vi "ECS - XNET CAN Interface.vi"() -> ()   [LabVIEW 2015, in "ECS-RT.lvlib"]
uses:
  ECS-RT.lvlib
  Typedefs/MISC/Control Parameters.ctl
  Globals/Calpoint IDs.vi
  <vilib>/xnet/xnet.llb/XNET String To IO Name (Database Alias).vi
  <vilib>/xnet/xnet.llb/XNET Database Close (Database).vi
  <vilib>/xnet/xnet.llb/XNET String To IO Name (Signal).vi
  <vilib>/xnet/xnet.llb/XNET Create Session (Signal Input Single-point).vi
  <vilib>/xnet/xnet.llb/XNET Read (Signal Single-point).vi
  <vilib>/xnet/xnet.llb/XNET Create Session (Signal Output Single-point).vi
  <vilib>/xnet/xnet.llb/XNET Write (Signal Single-point).vi
  <resource>/objmgr/xnet.rc
  <vilib>/addons/Software Calibration Management/_CalPointResources/scm32.dll
  ECS-Shared.lvlib
panel:
  out "XNET Control Params":T1[](array[typedef])
  in  "Wait":u32=2500 caption="[msec]"
  out "error out":errorcluster
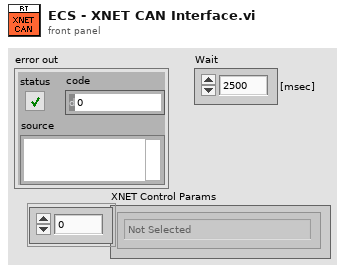
[diagram p1: front panel]
types:
  T1 = typedef "ECS-Shared.lvlib/Control Parameters.ctl" = enum16{"Not Selected", "Pedal Position [%]", "ESTOP", "Sensor1NOx", "Sensor1O2", "Sensor1SupplyStatus", "Sensor1TempStatus", "Sensor1NOxStatus", "Sensor1O2Status", "Sensor1HeaterMode", "Sensor1HeaterCircuit", "Sensor1NOxCircuit", "Sensor1O2Circuit", "Sensor2NOx", "Sensor2O2", "Sensor2SupplyStatus", "Sensor2TempStatus", "Sensor2NOxStatus", "Sensor2O2Status", "Sensor2HeaterMode", "Sensor2HeaterCircuit", "Sensor2NOxCircuit", "Sensor2O2Circuit"}
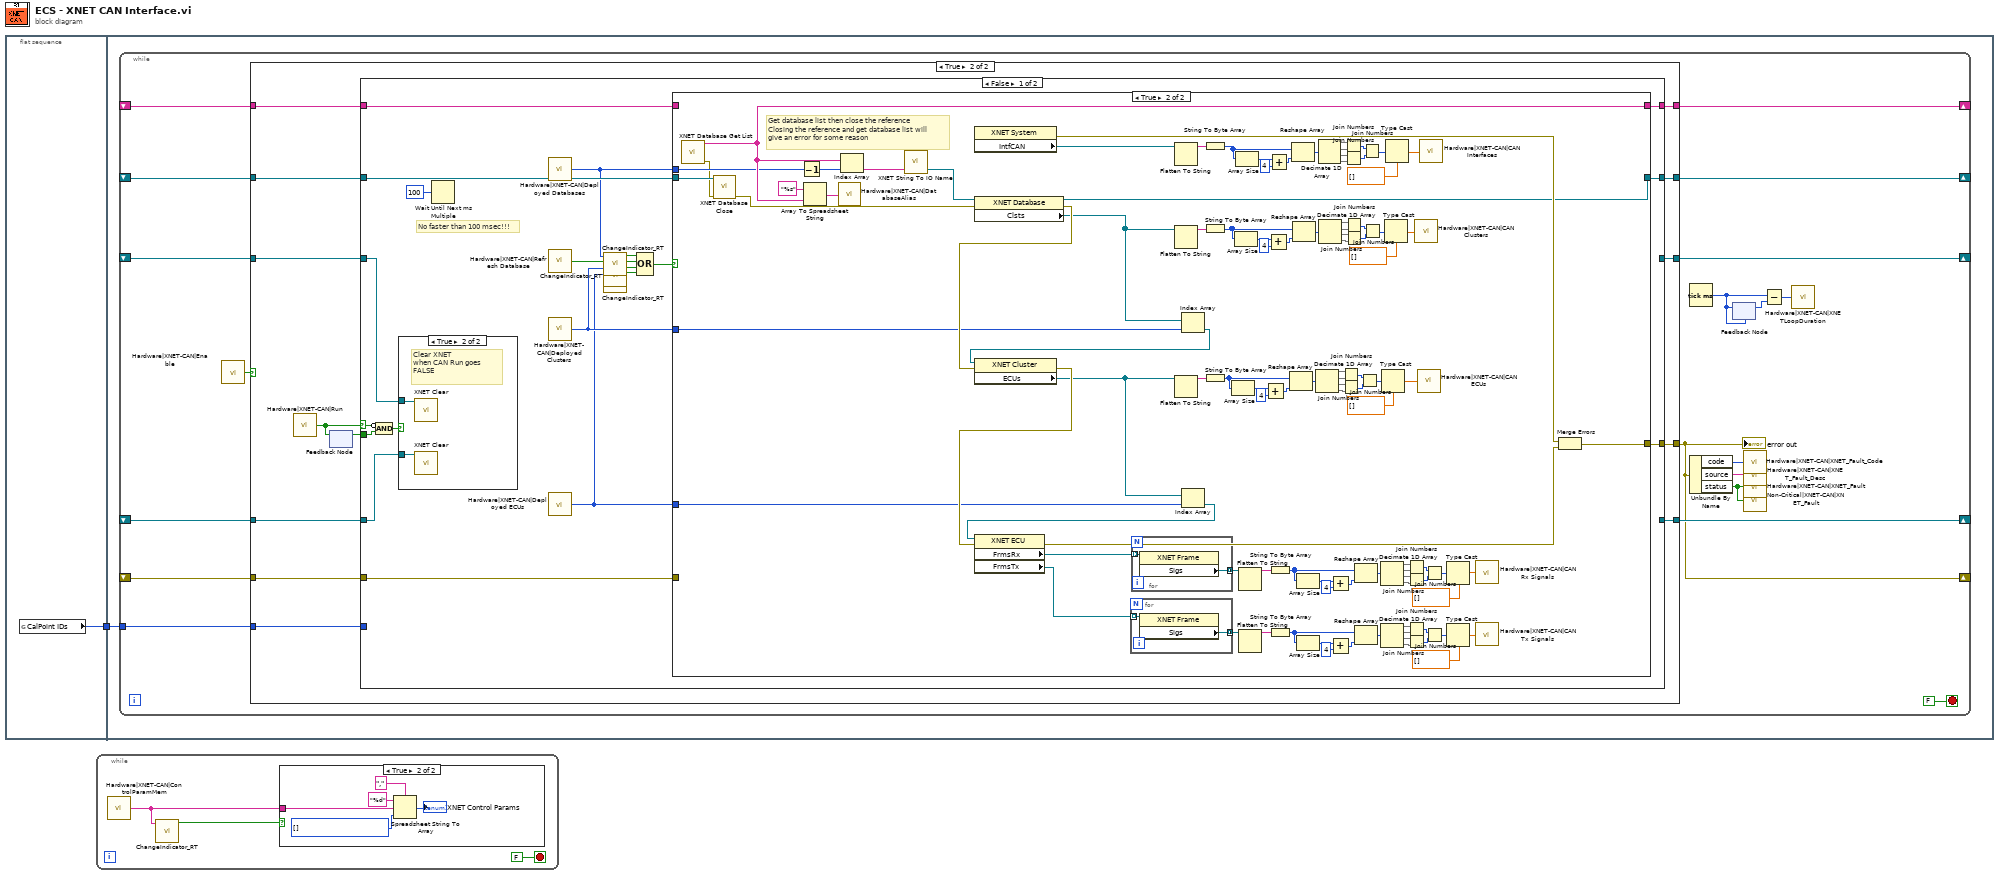
[diagram p0: block diagram]
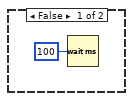
[diagram p2: hidden frame]
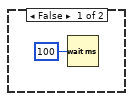
[diagram p3: hidden frame]
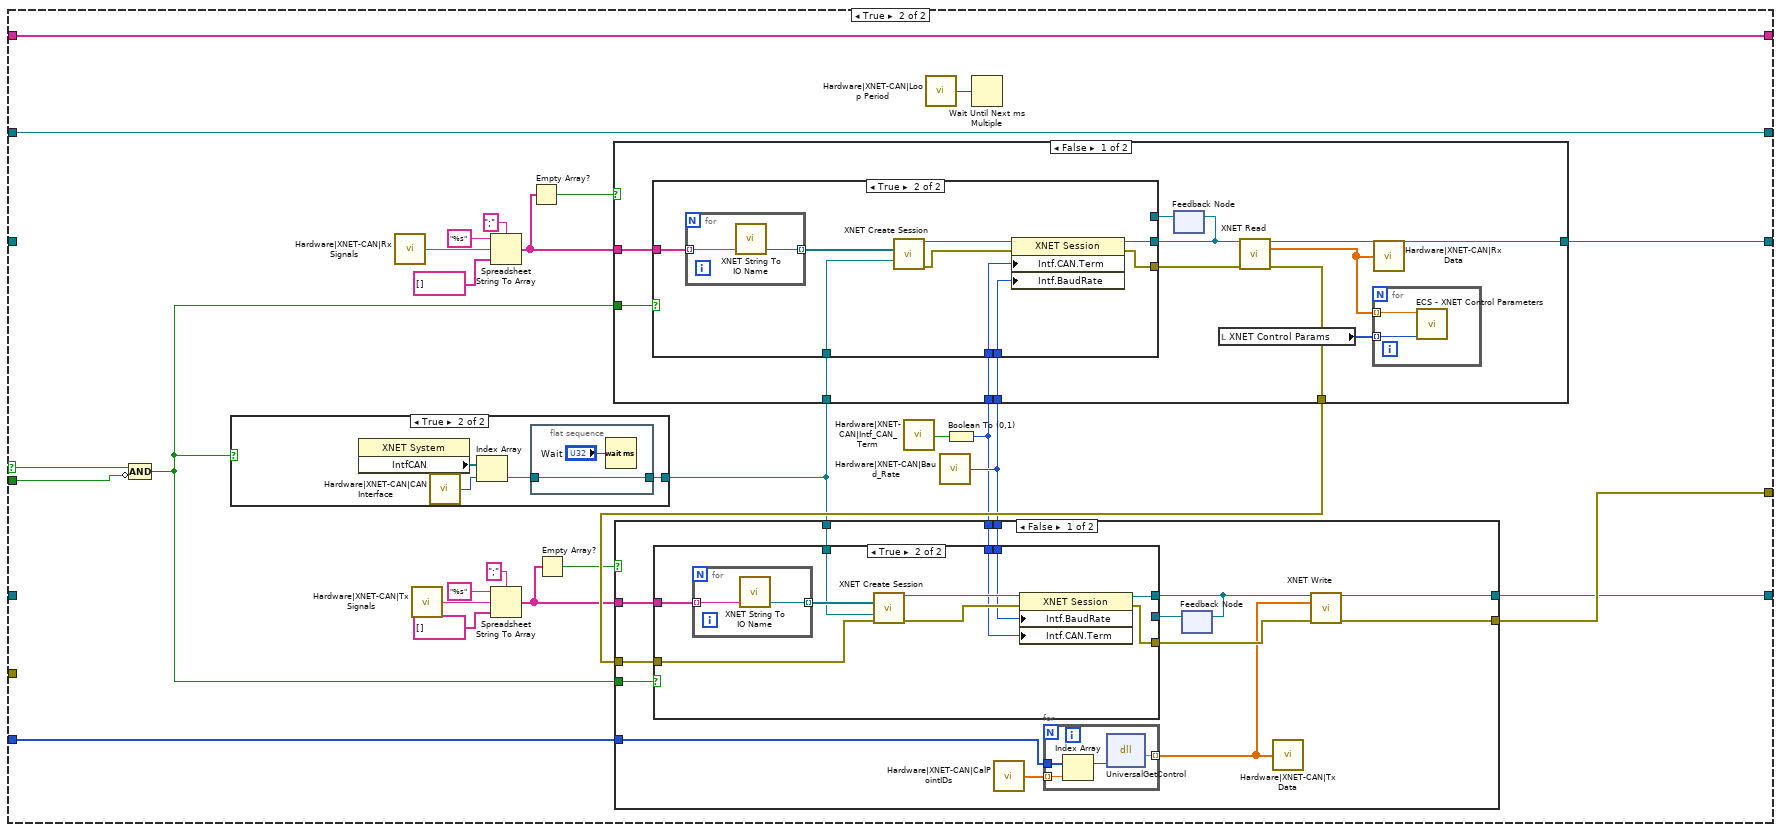
[diagram p6: hidden frame]
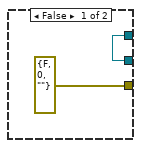
[diagram p8: hidden frame]
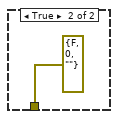
[diagram p9: hidden frame]
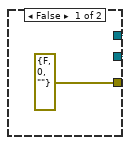
[diagram p10: hidden frame]
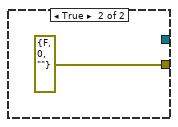
[diagram p11: hidden frame]
diagram:
  n1 = flat-sequence {
    tunnel: [w2] -> w1
    tunnel: w1 -> [w3]
    frame #0 {
      n2 = global read "Calpoint IDs.vi" "CalPoint IDs"() -> (w2:i32[])
    }
    frame #1 {
      n3 = while {
        shift-right: [w21] -> _
        shift-left: _ -> [w19]
        shift-right: [w22] -> _
        shift-left: _ -> [w20]
        shift-right: [w18] -> _
        shift-left: _ -> [w17]
        shift-right: [w11] -> _
        shift-left: _ -> [w10]
        shift-right: [w9] -> _
        shift-left: _ -> [w8]
        tunnel: w3 -> [w7]
        stop <- FALSE stop-if-true
        n4 = call "Hardware|XNET-CAN|Enable"() -> ("Value"=w4:bool)
        n5 = case shown="True" w4 {
          tunnel: [_ w34] -> w22
          tunnel: [_ w33] -> w21
          tunnel: w20 -> [_ w32]
          tunnel: w19 -> [_ w31]
          tunnel: [_ w30] -> w18
          tunnel: w17 -> [_ w29]
          tunnel: [_ w28] -> w11
          tunnel: w10 -> [_ w27]
          tunnel: [_ w26] -> w9
          tunnel: w8 -> [_ w25]
          tunnel: w7 -> [_ w24]
          frame False {
            n6 = Wait (ms)(milliseconds to wait=u32 100) -> ()  [unwired: 1 out]
          }
          frame True {
            n7 = call "Hardware|XNET-CAN|Run"() -> ("Value"=w36:bool)
            n8 = feedback #1() -> (w35:bool)  [unwired: 1 in]
            n9 = feedback-in #1(w36) -> ()
            n10 = case shown="False" w36 {
              selector: w36 -> [w56 w193]
              tunnel: [w51 w180] -> w26
              tunnel: w35 -> [w54 w171]
              tunnel: [_ w177] -> w34
              tunnel: [_ w176] -> w33
              tunnel: w32 -> [w53 _]
              tunnel: w31 -> [w52 _]
              tunnel: [w50 w173] -> w30
              tunnel: w29 -> [w48 w173]
              tunnel: [w49 w170] -> w28
              tunnel: w27 -> [w37 w170]
              tunnel: w25 -> [w38 _]
              tunnel: w24 -> [_ w168]
              frame False {
                # "No faster than 100 msec!!!"
                n11 = Compound Arithmetic op=AND(invert w56, w54) -> (w55:bool)
                n12 = case shown="True" w55 {
                  tunnel: w53 -> [_ w167]
                  tunnel: w52 -> [_ w166]
                  frame False {
                  }
                  frame True {
                    # "Clear XNET\nwhen CAN Run goes FALSE"
                    n13 = call <vilib>:"XNET Clear.vi"("session in"=w166) -> ()  [unwired: 14 in, 1 out]
                    n14 = call <vilib>:"XNET Clear.vi"("session in"=w167) -> ()  [unwired: 14 in, 1 out]
                  }
                }
                n15 = Wait Until Next ms Multiple(millisecond multiple=u32 100) -> ()  [unwired: 1 out]
                n16 = call "Hardware|XNET-CAN|Deployed Databases"() -> ("Value"=w44:i32)
                n17 = call "Hardware|XNET-CAN|Refresh Database"() -> ("Value"=w46:bool)
                n18 = call "Hardware|XNET-CAN|Deployed Clusters"() -> ("Value"=w41:i32)
                n19 = call "Hardware|XNET-CAN|Deployed ECUs"() -> ("Value"=w40:i32)
                n20 = call "ChangeIndicator_RT.vi"("Input"=w44) -> ("Change"=w45:bool)  [unwired: 9 in]
                n21 = call "ChangeIndicator_RT.vi"("Input"=w41) -> ("Change"=w43:bool)  [unwired: 9 in]
                n22 = call "ChangeIndicator_RT.vi"("Input"=w40) -> ("Change"=w42:bool)  [unwired: 9 in]
                n23 = Compound Arithmetic op=OR(w45, w46, w43, w42) -> (w39:bool)
                n24 = case shown="True" w39 {
                  tunnel: w40 -> [_ w159]
                  tunnel: [w59 w158] -> w51
                  tunnel: w41 -> [_ w151]
                  tunnel: [w57 w145] -> w50
                  tunnel: [w58 w144] -> w49
                  tunnel: w48 -> [w57 w143]
                  tunnel: w44 -> [_ w142]
                  tunnel: w38 -> [w59 _]
                  tunnel: w37 -> [w58 _]
                  frame False {
                  }
                  frame True {
                    # "Get database list then close the reference\nClosing the reference and get database list will\ngive an error for some reason"
                    n25 = call <vilib>:"XNET Database Get List.vi"() -> ("array of alias"=w144:string[], "error out"=w60:errorcluster)  [unwired: 13 in, 1 out]
                    n26 = call-poly <vilib>:"XNET Database Close.vi"("database in"=w143, "error in (no error)"=w60) -> ("error out"=w155:errorcluster)  [unwired: 13 in]
                    n27 = Decrement(x=w142) -> (x-1=w61:i32)
                    n28 = Array To Spreadsheet String(array=w144, 3:"%s" ("format string")) -> (spreadsheet string=w63:string)  [unwired: 1 in]
                    n29 = call "Hardware|XNET-CAN|DatabaseAlias"("Value"=w63) -> ()
                    n30 = Index Array(array=w144, index=w61) -> (element=w62:string)
                    n31 = call-poly <vilib>:"XNET String To IO Name.vi"("string"=w62) -> ("XNET Database"=w156:refnum<k21>)  [unwired: 4 out]
                    n32 = property class="XNET System"() -> (error out=w153:errorcluster, "IntfCAN"=w152:refnum<k21>[])  [unwired: 2 in, 1 out]
                    n33 = property class="XNET Database"(reference=w156, error in=w155) -> (reference out=w145:refnum<k21>, error out=w161:errorcluster, "Clsts"=w150:refnum<k21>[])
                    n34 = Flatten To String(anything=w152) -> (data string=w66:string)  [unwired: 3 in, 2 out]
                    n35 = Flatten To String(anything=w150) -> (data string=w81:string)  [unwired: 3 in, 2 out]
                    n36 = Index Array(array=w150, index=w151) -> (element=w149:refnum<k21>)
                    n37 = property class="XNET Cluster"(reference=w149, error in=w161) -> (error out=w160:errorcluster, "ECUs"=w148:refnum<k21>[])  [unwired: 1 out]
                    n38 = Flatten To String(anything=w148) -> (data string=w96:string)  [unwired: 3 in, 2 out]
                    n39 = Index Array(array=w148, index=w159) -> (element=w154:refnum<k21>)
                    n40 = property class="XNET ECU"(reference=w154, error in=w160) -> (error out=w157:errorcluster, "FrmsRx"=w147:refnum<k21>[], "FrmsTx"=w146:refnum<k21>[])  [unwired: 1 out]
                    n41 = for {
                      tunnel: w146 -> [w163] mode=indexing
                      tunnel: [w162] -> w110 mode=concatenating
                      n42 = property class="XNET Frame"(reference=w163) -> ("Sigs"=w162:refnum<k21>[])  [unwired: 1 in, 2 out]
                    }
                    n43 = for {
                      tunnel: w147 -> [w165] mode=indexing
                      tunnel: [w164] -> w111 mode=concatenating
                      n44 = property class="XNET Frame"(reference=w165) -> ("Sigs"=w164:refnum<k21>[])  [unwired: 1 in, 2 out]
                    }
                    n45 = String To Byte Array(string=w66) -> (unsigned byte array=w75:u8[])
                    n46 = String To Byte Array(string=w81) -> (unsigned byte array=w90:u8[])
                    n47 = String To Byte Array(string=w96) -> (unsigned byte array=w105:u8[])
                    n48 = Array Size(array=w105) -> (size(s)=w106:i32)
                    n49 = Array Size(array=w90) -> (size(s)=w91:i32)
                    n50 = Array Size(array=w75) -> (size(s)=w76:i32)
                    n51 = Flatten To String(anything=w111) -> (data string=w141:string)  [unwired: 3 in, 2 out]
                    n52 = Flatten To String(anything=w110) -> (data string=w112:string)  [unwired: 3 in, 2 out]
                    n53 = Add(x=w106, y=4) -> (x+y=w107:i32)
                    n54 = Add(x=w91, y=4) -> (x+y=w92:i32)
                    n55 = Add(x=w76, y=4) -> (x+y=w77:i32)
                    n56 = String To Byte Array(string=w141) -> (unsigned byte array=w132:u8[])
                    n57 = String To Byte Array(string=w112) -> (unsigned byte array=w121:u8[])
                    n58 = Reshape Array(w105, w107) -> (w104:u8[])
                    n59 = Reshape Array(w75, w77) -> (w74:u8[])
                    n60 = Reshape Array(w90, w92) -> (w89:u8[])
                    n61 = Array Size(array=w132) -> (size(s)=w131:i32)
                    n62 = Array Size(array=w121) -> (size(s)=w122:i32)
                    n63 = Decimate 1D Array(w104) -> (w109:u8[], w97:u8[], w98:u8[], w99:u8[])
                    n64 = Decimate 1D Array(w74) -> (w79:u8[], w67:u8[], w68:u8[], w69:u8[])
                    n65 = Decimate 1D Array(w89) -> (w94:u8[], w82:u8[], w83:u8[], w84:u8[])
                    n66 = Add(x=w131, y=4) -> (x+y=w130:i32)
                    n67 = Add(x=w122, y=4) -> (x+y=w123:i32)
                    n68 = Join Numbers(hi=w109, lo=w97) -> ((hi.lo)=w100:u16[])
                    n69 = Join Numbers(hi=w98, lo=w99) -> ((hi.lo)=w101:u16[])
                    n70 = Join Numbers(hi=w79, lo=w67) -> ((hi.lo)=w70:u16[])
                    n71 = Join Numbers(hi=w68, lo=w69) -> ((hi.lo)=w71:u16[])
                    n72 = Join Numbers(hi=w94, lo=w82) -> ((hi.lo)=w85:u16[])
                    n73 = Join Numbers(hi=w83, lo=w84) -> ((hi.lo)=w86:u16[])
                    n74 = Reshape Array(w132, w130) -> (w133:u8[])
                    n75 = Reshape Array(w121, w123) -> (w120:u8[])
                    n76 = Join Numbers(hi=w100, lo=w101) -> ((hi.lo)=w102:u32[])
                    n77 = Join Numbers(hi=w70, lo=w71) -> ((hi.lo)=w72:u32[])
                    n78 = Join Numbers(hi=w85, lo=w86) -> ((hi.lo)=w87:u32[])
                    n79 = Decimate 1D Array(w133) -> (w128:u8[], w140:u8[], w139:u8[], w138:u8[])
                    n80 = Decimate 1D Array(w120) -> (w125:u8[], w113:u8[], w114:u8[], w115:u8[])
                    n81 = Type Cast(type=sgl[] [], x=w102) -> (*(type *) &x=w95:sgl[])
                    n82 = Type Cast(type=sgl[] [], x=w87) -> (*(type *) &x=w80:sgl[])
                    n83 = Type Cast(type=sgl[] [], x=w72) -> (*(type *) &x=w65:sgl[])
                    n84 = Join Numbers(hi=w128, lo=w140) -> ((hi.lo)=w137:u16[])
                    n85 = Join Numbers(hi=w139, lo=w138) -> ((hi.lo)=w136:u16[])
                    n86 = Join Numbers(hi=w125, lo=w113) -> ((hi.lo)=w116:u16[])
                    n87 = Join Numbers(hi=w114, lo=w115) -> ((hi.lo)=w117:u16[])
                    n88 = call "Hardware|XNET-CAN|CAN Clusters"("Value"=w80) -> ()
                    n89 = call "Hardware|XNET-CAN|CAN ECUs"("Value"=w95) -> ()
                    n90 = call "Hardware|XNET-CAN|CAN Interfaces"("Value"=w65) -> ()
                    n91 = Join Numbers(hi=w137, lo=w136) -> ((hi.lo)=w135:u32[])
                    n92 = Join Numbers(hi=w116, lo=w117) -> ((hi.lo)=w118:u32[])
                    n93 = Type Cast(type=sgl[] [], x=w135) -> (*(type *) &x=w127:sgl[])
                    n94 = Type Cast(type=sgl[] [], x=w118) -> (*(type *) &x=w126:sgl[])
                    n95 = call "Hardware|XNET-CAN|CAN Rx Signals"("Value"=w127) -> ()
                    n96 = call "Hardware|XNET-CAN|CAN Tx Signals"("Value"=w126) -> ()
                    n97 = Merge Errors(w153, w157) -> (w158:errorcluster)
                  }
                }
              }
              frame True {
                n98 = Compound Arithmetic op=AND(w193, invert w171) -> (w172:bool)
                n99 = case shown="True" w172 {
                  tunnel: [_ w195] -> w181
                  frame False {
                  }
                  frame True {
                    n100 = property class="XNET System"() -> ("IntfCAN"=w197:refnum<k21>[])  [unwired: 2 in, 2 out]
                    n101 = call "Hardware|XNET-CAN|CAN Interface"() -> ("Value"=w198:u8)
                    n102 = Index Array(array=w197, index=w198) -> (element=w196:refnum<k21>)
                    n103 = flat-sequence {
                      tunnel: w196 -> [w199]
                      tunnel: [w199] -> w195
                      frame #0 {
                        n104 = Wait (ms)(milliseconds to wait="Wait") -> ()  [unwired: 1 out]
                      }
                    }
                  }
                }
                n105 = call "Hardware|XNET-CAN|Rx Signals"() -> ("Value"=w184:string)
                n106 = call "Hardware|XNET-CAN|Tx Signals"() -> ("Value"=w191:string)
                n107 = Spreadsheet String To Array(delimiter (Tab)=";", format string="%s", spreadsheet string=w184, array type (2D Dbl)=string[] [] ("CAN Signals 2")) -> (array=w182:string[])
                n108 = Spreadsheet String To Array(delimiter (Tab)=";", format string="%s", spreadsheet string=w191, array type (2D Dbl)=string[] [] ("CAN Signals 2")) -> (array=w188:string[])
                n109 = Empty Array?(array=w182) -> (empty?=w183:bool)
                n110 = Empty Array?(array=w188) -> (empty?=w189:bool)
                n111 = call "Hardware|XNET-CAN|Intf_CAN_Term"() -> ("Value"=w175:bool)
                n112 = call "Hardware|XNET-CAN|Loop Period"() -> ("Value"=w169:u32)
                n113 = call "Hardware|XNET-CAN|Baud_Rate"() -> ("Value"=w187:u32)
                n114 = Boolean To (0,1)(Boolean=w175) -> (0, 1=w174:i16)
                n115 = case shown="False" w183 {
                  tunnel: w187 -> [w212 _]
                  tunnel: w172 -> [w208 _]
                  tunnel: w182 -> [w207 _]
                  tunnel: w181 -> [w206 _]
                  tunnel: [w205 errorcluster {"status"=FALSE, "code"=0, "source"=""} ("error out")] -> w194
                  tunnel: [w204 _] -> w176
                  tunnel: w174 -> [w203 _]
                  frame False {
                    n116 = feedback #2() -> (w209:refnum<k21>)  [unwired: 1 in]
                    n117 = case shown="True" w208 {
                      tunnel: w212 -> [_ w223]
                      tunnel: [errorcluster {"status"=FALSE, "code"=0, "source"=""} ("error out") w222] -> w211
                      tunnel: [w216 w221] -> w210
                      tunnel: w209 -> [w216 _]
                      tunnel: w207 -> [_ w220]
                      tunnel: w206 -> [_ w219]
                      tunnel: w203 -> [_ w217]
                      frame False {
                      }
                      frame True {
                        n118 = for {
                          tunnel: [w226] -> w225 mode=indexing
                          tunnel: w220 -> [w227] mode=indexing
                          n119 = call-poly <vilib>:"XNET String To IO Name.vi"("string"=w227) -> ("XNET Signal"=w226:refnum<k21>)  [unwired: 4 out]
                        }
                        n120 = call-poly <vilib>:"XNET Create Session.vi"("signal list"=w225, "interface"=w219) -> ("session out"=w224:refnum<k21>, "error out"=w218:errorcluster)  [unwired: 1 in, 11 out]
                        n121 = property class="XNET Session"(reference=w224, error in=w218, "Intf.CAN.Term"=w217, "Intf.BaudRate"=w223) -> (reference out=w221:refnum<k21>, error out=w222:errorcluster)
                      }
                    }
                    n122 = feedback-in #2(w210) -> ()
                    n123 = local read "XNET Control Params"() -> (w202:T1[])
                    n124 = call-poly <vilib>:"XNET Read.vi"("session in"=w210, "error in (no error)"=w211) -> ("session out"=w204:refnum<k21>, "data"=w201:dbl[], "error out"=w205:errorcluster)  [unwired: 11 in]
                    n125 = for {
                      tunnel: w202 -> [w213] mode=indexing
                      tunnel: w201 -> [w214] mode=indexing
                      n126 = call "ECS - XNET Control Parameters.vi"("XNET Control Parameters"=w213, "Rx Data"=w214) -> ()  [unwired: 10 in]
                    }
                    n127 = call "Hardware|XNET-CAN|Rx Data"("Value"=w201) -> ()
                  }
                  frame True {
                  }
                }
                n128 = case shown="False" w189 {
                  tunnel: [w241 errorcluster {"status"=FALSE, "code"=0, "source"=""} ("error out")] -> w180
                  tunnel: w172 -> [w239 _]
                  tunnel: w188 -> [w238 _]
                  tunnel: w187 -> [w237 _]
                  tunnel: w181 -> [w235 _]
                  tunnel: w194 -> [w234 _]
                  tunnel: [w233 _] -> w177
                  tunnel: w174 -> [w232 _]
                  tunnel: w168 -> [w229 _]
                  frame False {
                    n129 = call "Hardware|XNET-CAN|CalPointIDs"() -> ("Value"=w231:sgl[])
                    n130 = for {
                      tunnel: w229 -> [w246]
                      tunnel: [w245] -> w230 mode=indexing
                      tunnel: w231 -> [w243] mode=indexing
                      n131 = Index Array(array=w246, index=w243) -> (element=w244:i32)
                      n132 = dll-call lib="C:/Program Files (x86)/National Instruments/LabVIEW 2015/vi.lib/addons/Software Calibration Management/_CalPointResources/scm*.*" fn="UniversalGetControl"("ID"=w244) -> ("return type"=w245:sgl)  [unwired: 4 in, 2 out]
                    }
                    n133 = feedback #3() -> (w240:refnum<k21>)  [unwired: 1 in]
                    n134 = case shown="True" w239 {
                      tunnel: [w248 w256] -> w242
                      tunnel: w240 -> [w248 _]
                      tunnel: [errorcluster {"status"=FALSE, "code"=0, "source"=""} ("error out") w254] -> w236
                      tunnel: w237 -> [_ w253]
                      tunnel: w238 -> [_ w252]
                      tunnel: w235 -> [_ w251]
                      tunnel: w234 -> [_ w250]
                      tunnel: w232 -> [_ w249]
                      frame False {
                      }
                      frame True {
                        n135 = for {
                          tunnel: [w259] -> w258 mode=indexing
                          tunnel: w252 -> [w260] mode=indexing
                          n136 = call-poly <vilib>:"XNET String To IO Name.vi"("string"=w260) -> ("XNET Signal"=w259:refnum<k21>)  [unwired: 4 out]
                        }
                        n137 = call-poly <vilib>:"XNET Create Session.vi"("signal list"=w258, "interface"=w251, "error in (no error)"=w250) -> ("session out"=w257:refnum<k21>, "error out"=w255:errorcluster)  [unwired: 11 out]
                        n138 = property class="XNET Session"(reference=w257, error in=w255, "Intf.BaudRate"=w253, "Intf.CAN.Term"=w249) -> (reference out=w256:refnum<k21>, error out=w254:errorcluster)
                      }
                    }
                    n139 = feedback-in #3(w242) -> ()
                    n140 = call "Hardware|XNET-CAN|Tx Data"("Value"=w230) -> ()
                    n141 = call-poly <vilib>:"XNET Write.vi"("session in"=w242, "data"=w230, "error in (no error)"=w236) -> ("session out"=w233:refnum<k21>, "error out"=w241:errorcluster)  [unwired: 11 in]
                  }
                  frame True {
                  }
                }
                n142 = Wait Until Next ms Multiple(millisecond multiple=w169) -> ()  [unwired: 1 out]
              }
            }
          }
        }
        "error out" <- w9
        n143 = Tick Count (ms)() -> (millisecond timer value=w5:u32)
        n144 = Unbundle By Name(w9) -> ("code"=w16:i32, "source"=w12:string, "status"=w13:bool)
        n145 = feedback-in #4(w5) -> ()
        n146 = feedback #4(w5) -> (w15:u32)
        n147 = call "Hardware|XNET-CAN|XNET_Fault_Code"("Value"=w16) -> ()
        n148 = call "Hardware|XNET-CAN|XNET_Fault_Desc"("Value"=w12) -> ()
        n149 = call "Hardware|XNET-CAN|XNET_Fault"("Value"=w13) -> ()
        n150 = call "Non-Critical|XNET-CAN|XNET_Fault"("Fault"=w13) -> ()  [unwired: 2 in]
        n151 = Subtract(x=w5, y=w15) -> (x-y=w14:u32)
        n152 = call "Hardware|XNET-CAN|XNETLoopDuration"("Value"=w14) -> ()
      }
    }
  }
  n153 = while {
    stop <- FALSE stop-if-true
    n154 = call "Hardware|XNET-CAN|ControlParamMem"() -> ("Value"=w263:string)
    n155 = call "ChangeIndicator_RT.vi"("Input"=w263) -> ("Change"=w264:bool)  [unwired: 9 in]
    n156 = case shown="True" w264 {
      tunnel: w263 -> [_ w268]
      frame False {
        n157 = Wait (ms)(milliseconds to wait=u32 100) -> ()  [unwired: 1 out]
      }
      frame True {
        w267 = T1[] [] items=["Not Selected", "Pedal Position [%]", "ESTOP", "Sensor1NOx", "Sensor1O2", "Sensor1SupplyStatus", "Sensor1TempStatus", "Sensor1NOxStatus", "Sensor1O2Status", "Sensor1HeaterMode", "Sensor1HeaterCircuit", "Sensor1NOxCircuit", "Sensor1O2Circuit", "Sensor2NOx", "Sensor2O2", "Sensor2SupplyStatus", "Sensor2TempStatus", "Sensor2NOxStatus", "Sensor2O2Status", "Sensor2HeaterMode", "Sensor2HeaterCircuit", "Sensor2NOxCircuit", "Sensor2O2Circuit"]
        n158 = Spreadsheet String To Array(delimiter (Tab)=",", format string="%d", spreadsheet string=w268, array type (2D Dbl)=w267) -> (array=→"XNET Control Params":T1[])
      }
    }
  }
